vi "Write channel active (index).vi"(8 "error in (no error)":errorcluster, 10 "channel active (index)":i32, 11 "OSA300 in":refnum<class "OSA300.lvclass">) -> (0 "error out":errorcluster, 3 "OSA300 out":refnum<class "OSA300.lvclass">)   [LabVIEW 2010, in "OSA300.lvclass"]
uses:
  OSA300.lvclass
  OSA300.lvclass/OSA300.ctl
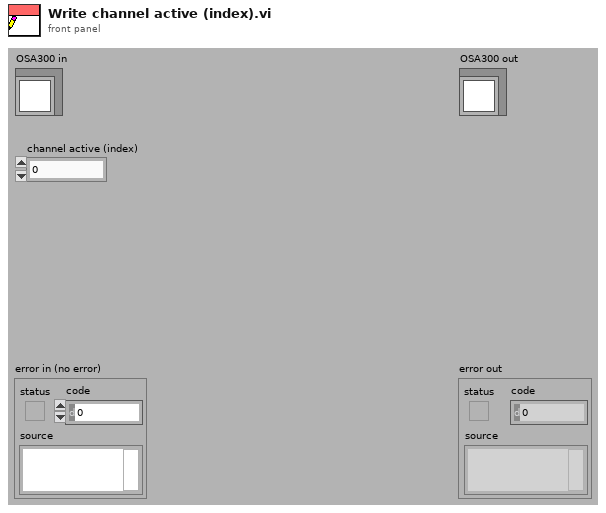
[diagram p1: front panel]
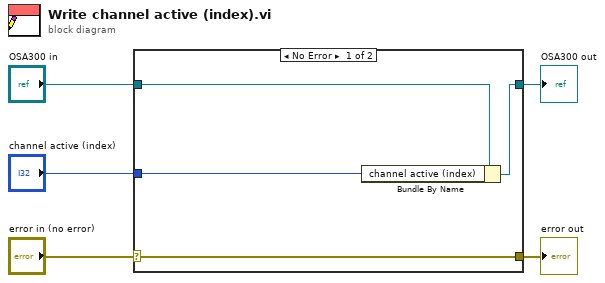
[diagram p0: block diagram]
diagram:
  n1 = case shown="No Error" "error in (no error)" {
    selector: "error in (no error)" -> [w9 w10]
    tunnel: [w9 w10] -> w4
    tunnel: [w7 w11] -> w2
    tunnel: "OSA300 in" -> [w8 w11]
    tunnel: "channel active (index)" -> [w6 _]
    frame No Error {
      n2 = Bundle By Name(cluster=w8, "channel active (index)"=w6) -> (w7:refnum<class "OSA300.lvclass">)
    }
    frame Error {
    }
  }
  "error out" <- w4
  "OSA300 out" <- w2
